vi "AutofocusScan.vi"() -> ()   [LabVIEW 2019]
uses:
  <vilib>/userDefined/High Color/IMAQdx.ctl
  <vilib>/vision/NI_Vision_Development_Module.lvlib
panel:
  out "MaxVal":dbl
  out "BestZ":dbl
  out "SDvsZ":string
  out "Sobel_SD":picture
  in  "Z OutputFile":path=path "C:/Users/TTUHEP/Documents/LabVIEW/GantryPrograms/Configs/temp.txt"
  in  "Plot Output File":string="C:\\Users\\TTUHEP\\Documents\\LabVIEW\\GantryPrograms\\LogFiles\\plot.png"
  out "spreadsheet string":string
  out "AfterFilter":T1(plugin-control)
  out "Image":T1(plugin-control)
  in  "Steps":dbl=20.0
  in  "ScanRange":dbl=0.2
  out "error out":errorcluster
  in  "error in (no error)":errorcluster
  in  "Z":dbl=68.166
  in  "Y":dbl=999.797
  in  "X":dbl=227.948
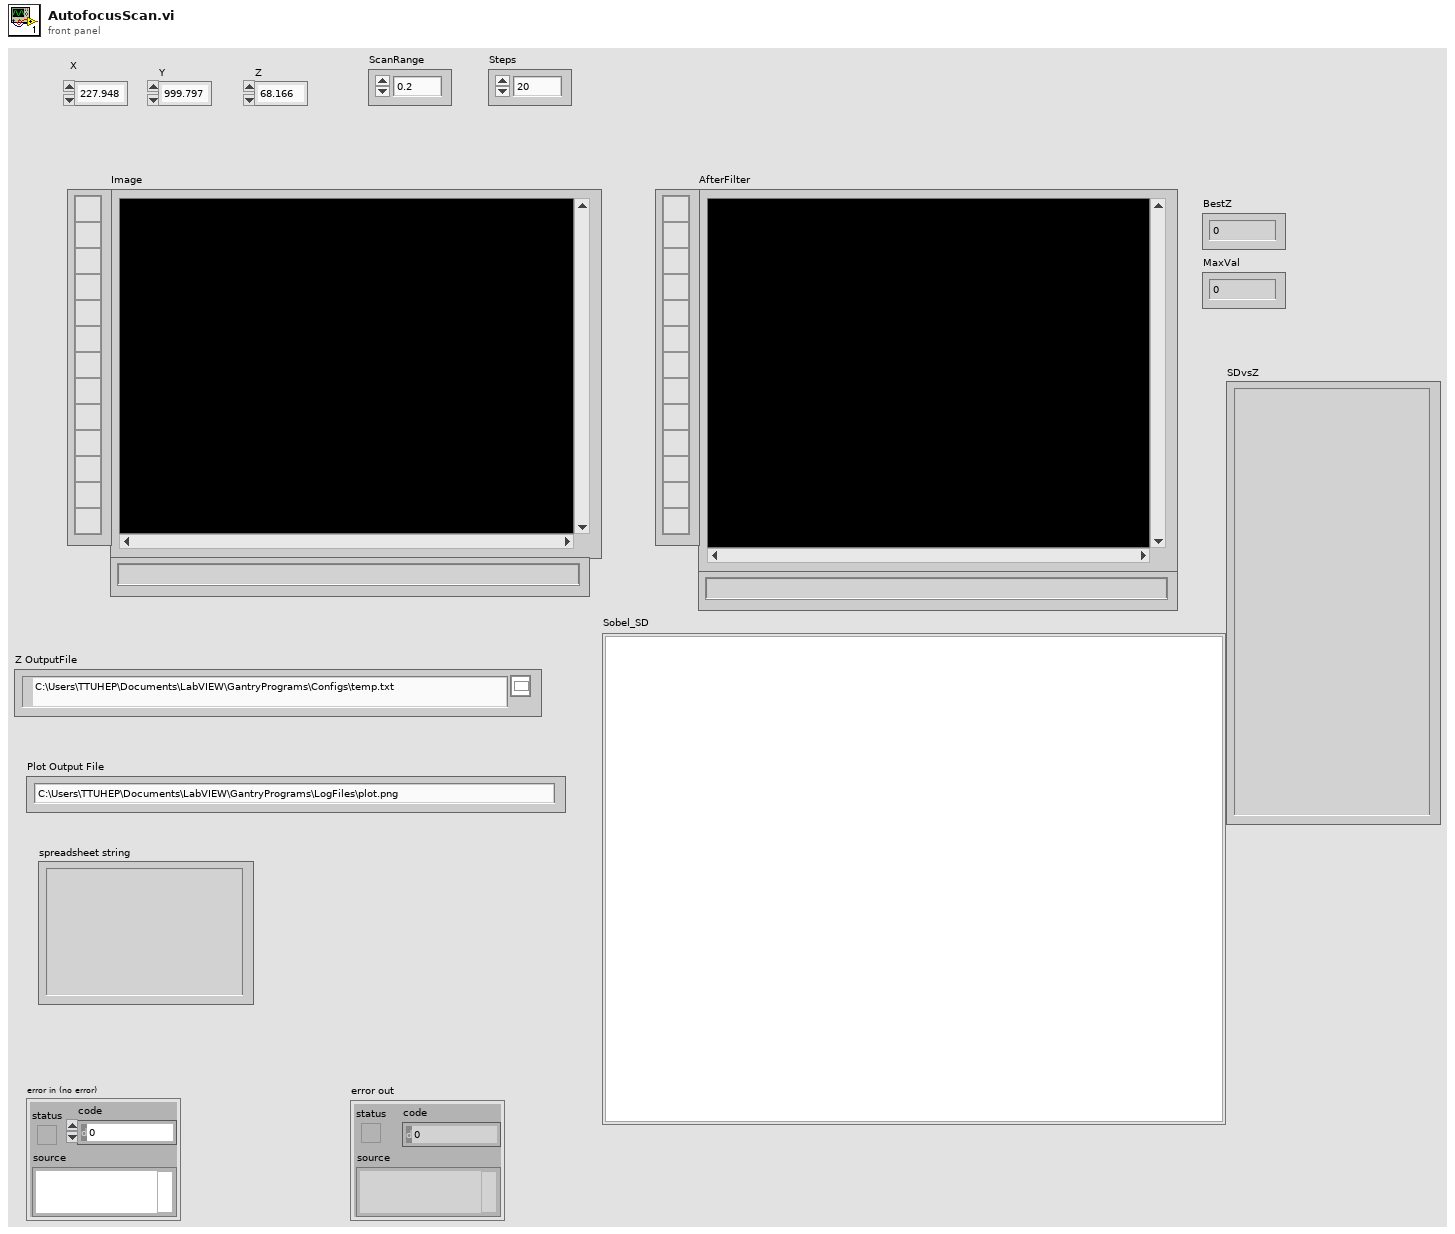
[diagram p1: front panel]
types:
  T1 = typedef "IMAQ Image.ctl" = refnum<image>
  T2 = enum16{"open", "replace", "create", "open or create", "replace or create", "replace or create with confirmation"}
  T3 = enum32{"Differentiation", "Gradient", "Prewitt", "Roberts", "Sigma", "Sobel"}
  T4 = typedef "IMAQdx.ctl" = refnum<k21>
  T5 = typedef "Image Type" = u32
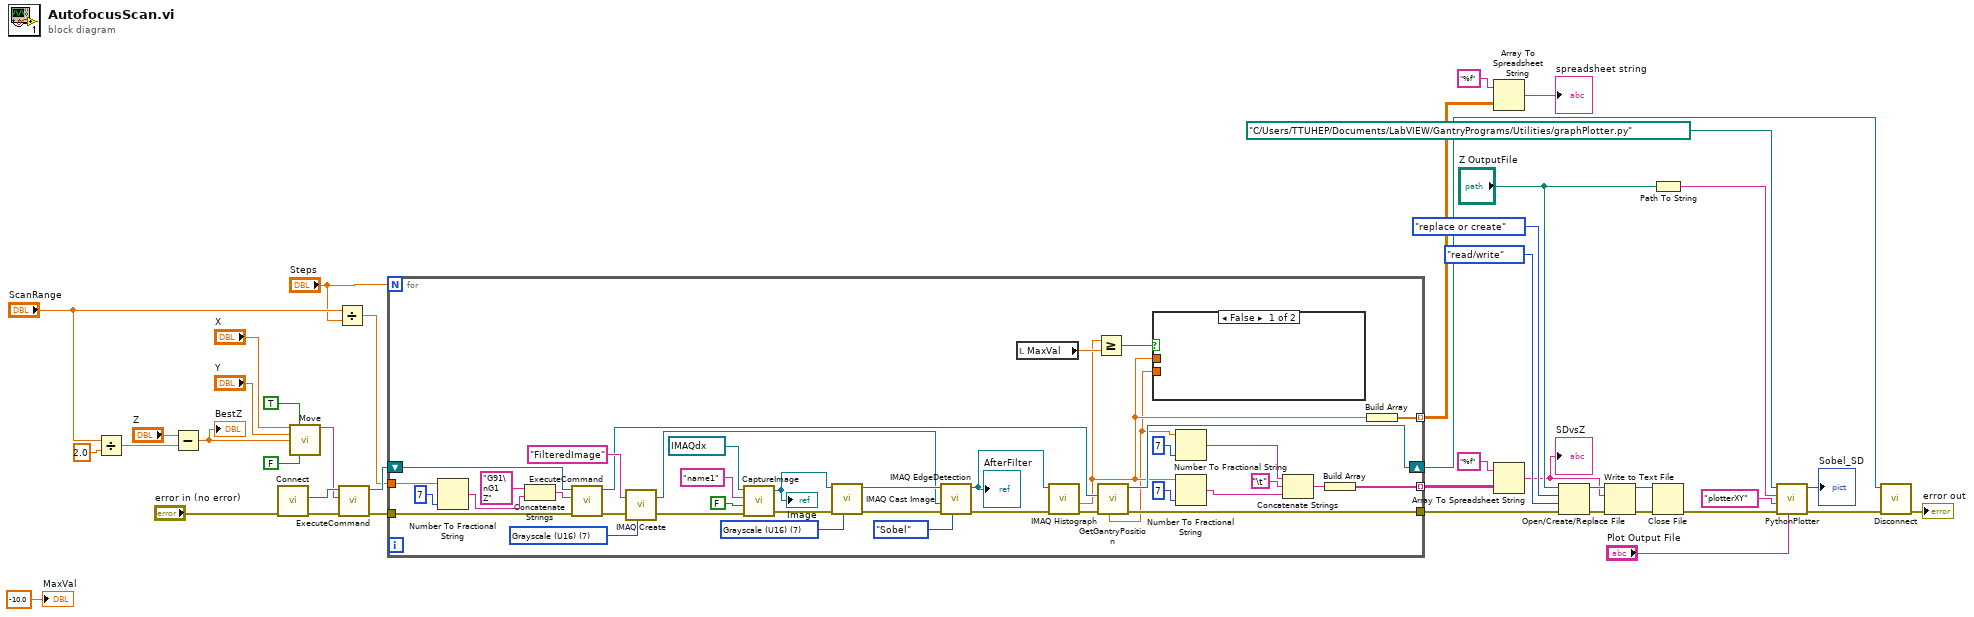
[diagram p0: block diagram]
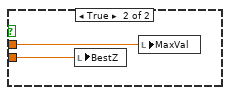
[diagram p2: hidden frame]
diagram:
  n1 = Divide(x="ScanRange", y=2.0) -> (x/y=w39:dbl)
  n2 = Subtract(x="Z", y=w39) -> (x-y=w2:dbl)
  "BestZ" <- w2
  n3 = call "Connect.vi"("error in (no error)"="error in (no error)") -> ("error out"=w31:errorcluster, "controller"=w33:refnum<k24>)  [unwired: 9 in]
  n4 = call "Move.vi"("X"="X", "Absolute"=TRUE, "Y"="Y", "Z"=w2, "Move Z first"=FALSE) -> ("Position Gcode"=w32:string)  [unwired: 10 in]
  n5 = Divide(x="ScanRange", y="Steps") -> (x/y=w26:dbl)
  n6 = call "ExecuteCommand.vi"("error in (no error)"=w31, "Command Code"=w32, "controller in"=w33) -> ("error out"=w30:errorcluster, "controller out"=w29:refnum<k24>)  [unwired: 6 in, 1 out]
  n7 = for {
    N: "Steps" -> [_]
    tunnel: w30 -> [w59]
    tunnel: w26 -> [w64]
    shift-right: [w53] -> w25
    shift-left: w29 -> [w65]
    tunnel: [w55] -> w10
    tunnel: [w54] -> w9 mode=indexing
    tunnel: [w48] -> w5 mode=indexing
    w67 = T5 7 items=["Grayscale (U8)", "Grayscale (I16)", "Grayscale (SGL)", "Complex (CSG)", "RGB (U32)", "HSL (U32)", "RGB (U64)", "Grayscale (U16)"] ("Image Type")
    w72 = T5 7 items=["Grayscale (U8)", "Grayscale (I16)", "Grayscale (SGL)", "Complex (CSG)", "RGB (U32)", "HSL (U32)", "RGB (U64)", "Grayscale (U16)"] ("Image Type")
    n8 = Number To Fractional String(number=w64, precision (6)=i16 7) -> (F-format string=w61:string)  [unwired: 2 in]
    n9 = Concatenate Strings("G91\nG1 Z", w61) -> (w60:string)
    n10 = call "ExecuteCommand.vi"("error in (no error)"=w59, "Command Code"=w60, "controller in"=w65) -> ("error out"=w58:errorcluster, "controller out"=w57:refnum<k24>)  [unwired: 6 in, 1 out]
    n11 = call "IMAQ Create"("Image Name"="FilteredImage", "Image Type"=w67, "error in (no error)"=w58) -> ("New Image"=w68:T1, "error out"=w77:errorcluster)  [unwired: 2 in]
    n12 = call "CaptureImage.vi"("Camera"=T4 "cam1", "ImageName"="name1", "Draw50MicroCircleAtCenter"=FALSE, "error in (no error)"=w77) -> ("Image"=w76:T1, "error out"=w75:errorcluster)  [unwired: 3 in]
    "Image" <- w76
    n13 = call "IMAQ Cast Image"("Image Type"=w72, "error in (no error)"=w75, "Image Src"=w76) -> ("error out"=w74:errorcluster, "Image Dst Out"=w73:T1)  [unwired: 7 in]
    n14 = call "IMAQ EdgeDetection"("Method"=T3."Sobel", "error in (no error)"=w74, "Image Dst"=w68, "Image Src"=w73) -> ("error out"=w71:errorcluster, "Image Dst Out"=w70:T1)  [unwired: 6 in]
    "AfterFilter" <- w70
    n15 = local read "MaxVal"() -> (w45:dbl)
    n16 = call "IMAQ Histograph"("error in (no error)"=w71, "Image"=w70) -> ("error out"=w56:errorcluster, "Standard  Deviation"=w43:sgl)  [unwired: 6 in, 2 out]
    n17 = Greater Or Equal?(x=w43, y=w45) -> (x >= y?=w44:bool)
    n18 = call "GetGantryPosition.vi"("error in (no error)"=w56, "Controller In"=w57) -> ("error out"=w55:errorcluster, "controller out"=w53:refnum<k24>, "Position Z"=w42:dbl)  [unwired: 3 in, 4 out]
    n19 = case shown="False" w44 {
      tunnel: w43 -> [_ w82]
      tunnel: w42 -> [_ w81]
      frame False {
      }
      frame True {
        n20 = local write "BestZ"(w81) -> ()
        n21 = local write "MaxVal"(w82) -> ()
      }
    }
    n22 = Number To Fractional String(number=w42, precision (6)=i16 7) -> (F-format string=w47:string)  [unwired: 2 in]
    n23 = Number To Fractional String(number=w43, precision (6)=i16 7) -> (F-format string=w46:string)  [unwired: 2 in]
    n24 = Concatenate Strings(w47, "\t", w46) -> (w49:string)
    n25 = Build Array(w49) -> (w48:string[])
    n26 = Build Array(w43) -> (w54:sgl[])
  }
  n27 = Array To Spreadsheet String(array=w9, 3:"%f" ("format string")) -> (spreadsheet string=→"spreadsheet string":string)  [unwired: 1 in]
  n28 = Array To Spreadsheet String(array=w5, 3:"%f" ("format string")) -> (spreadsheet string=w3:string)  [unwired: 1 in]
  "SDvsZ" <- w3
  n29 = Open/Create/Replace File(file path (use dialog)="Z OutputFile", error in=w10, operation (0:open)=T2."replace or create", access (0:read/write)=enum16{"read/write", "read-only", "write-only"}."read/write") -> (refnum out=w18:refnum<file>, error out=w19:errorcluster)  [unwired: 2 in, 1 out]
  n30 = Write to Text File(file (use dialog)=w18, text=w3, error in=w19) -> (refnum out=w21:refnum<file>, error out=w20:errorcluster)  [unwired: 1 in, 1 out]
  n31 = Path To String(path="Z OutputFile") -> (string=w13:string)
  n32 = Close File(refnum=w21, error in=w20) -> (error out=w12:errorcluster)  [unwired: 1 out]
  n33 = call "PythonPlotter.vi"("Output File"="Plot Output File", "error in (no error)"=w12, "Function Name"="plotterXY", "Input File"=w13, "Python Path"=path "C:/Users/TTUHEP/Documents/LabVIEW/GantryPrograms/Utilities/graphPlotter.py") -> ("error out"=w7:errorcluster, "HighVSPosition"=→"Sobel_SD":picture)  [unwired: 4 in]
  n34 = call "Disconnect.vi"("error in (no error)"=w7, "controller"=w25) -> ("error out"=→"error out":errorcluster)  [unwired: 9 in]
  "MaxVal" <- -10.0 ("MaxVal")
